vi "Main.vi"() -> ()   [LabVIEW 2018]
uses:
  <vilib>/myRIO/Instrument Drivers/Onboard IO/AI/vis/Read.vi
  <vilib>/myRIO/Common/Instrument Driver Framework/myRIO v1.0/UART/vis/myRIO v1.0 Close UART.vi
  <vilib>/myRIO/Instrument Drivers/Onboard IO/AI/vis/Smart Open.vi
  <vilib>/Utility/error.llb/Error Cluster From Error Code.vi
  <vilib>/myRIO/Common/Instrument Driver Framework/myRIO v1.0/AI/vis/myRIO v1.0 Read AI.vi
  <vilib>/myRIO/Common/Instrument Driver Framework/Utilities/vis/FPGA Ref Manager.vi
  <vilib>/myRIO/Common/Instrument Driver Framework/myRIO v1.0/myRIO v1.0 Reset FPGA.vi
  <vilib>/myRIO/Common/Instrument Driver Framework/myRIO v1.0/IRQ/vis/myRIO v1.0 IRQ Info FGV.vi
  <vilib>/myRIO/Common/Instrument Driver Framework/myRIO v1.0/IRQ/vis/myRIO v1.0 Timer IRQ Info FGV.vi
  <vilib>/myRIO/Common/Instrument Driver Framework/myRIO v1.0/IRQ/vis/myRIO v1.0 ISR Agent.vi
  <vilib>/myRIO/Instrument Drivers/Utilities/Utilities.lvlib
  <vilib>/ptbypt/NI_PtbyPt.lvlib
panel:
  out "웨이브폼 차트":dbl(graph)
  out "범위 밖":bool
  out "numeric":dbl format="%_3g"
  in  "Koffset [cm]":dbl
  in  "Kscale [cm-V]":dbl=27.5
  out "Vo [V]":dbl format="%.2f"
  out "Range [cm]":dbl(knob) scale=0.0..80.0
  in  "[ESC]":bool
  # "IR Range Finder demo"
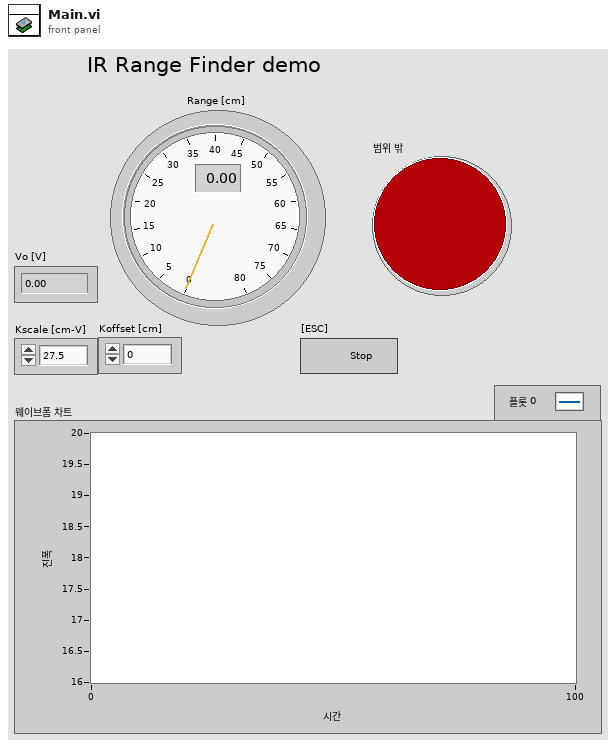
[diagram p1: front panel]
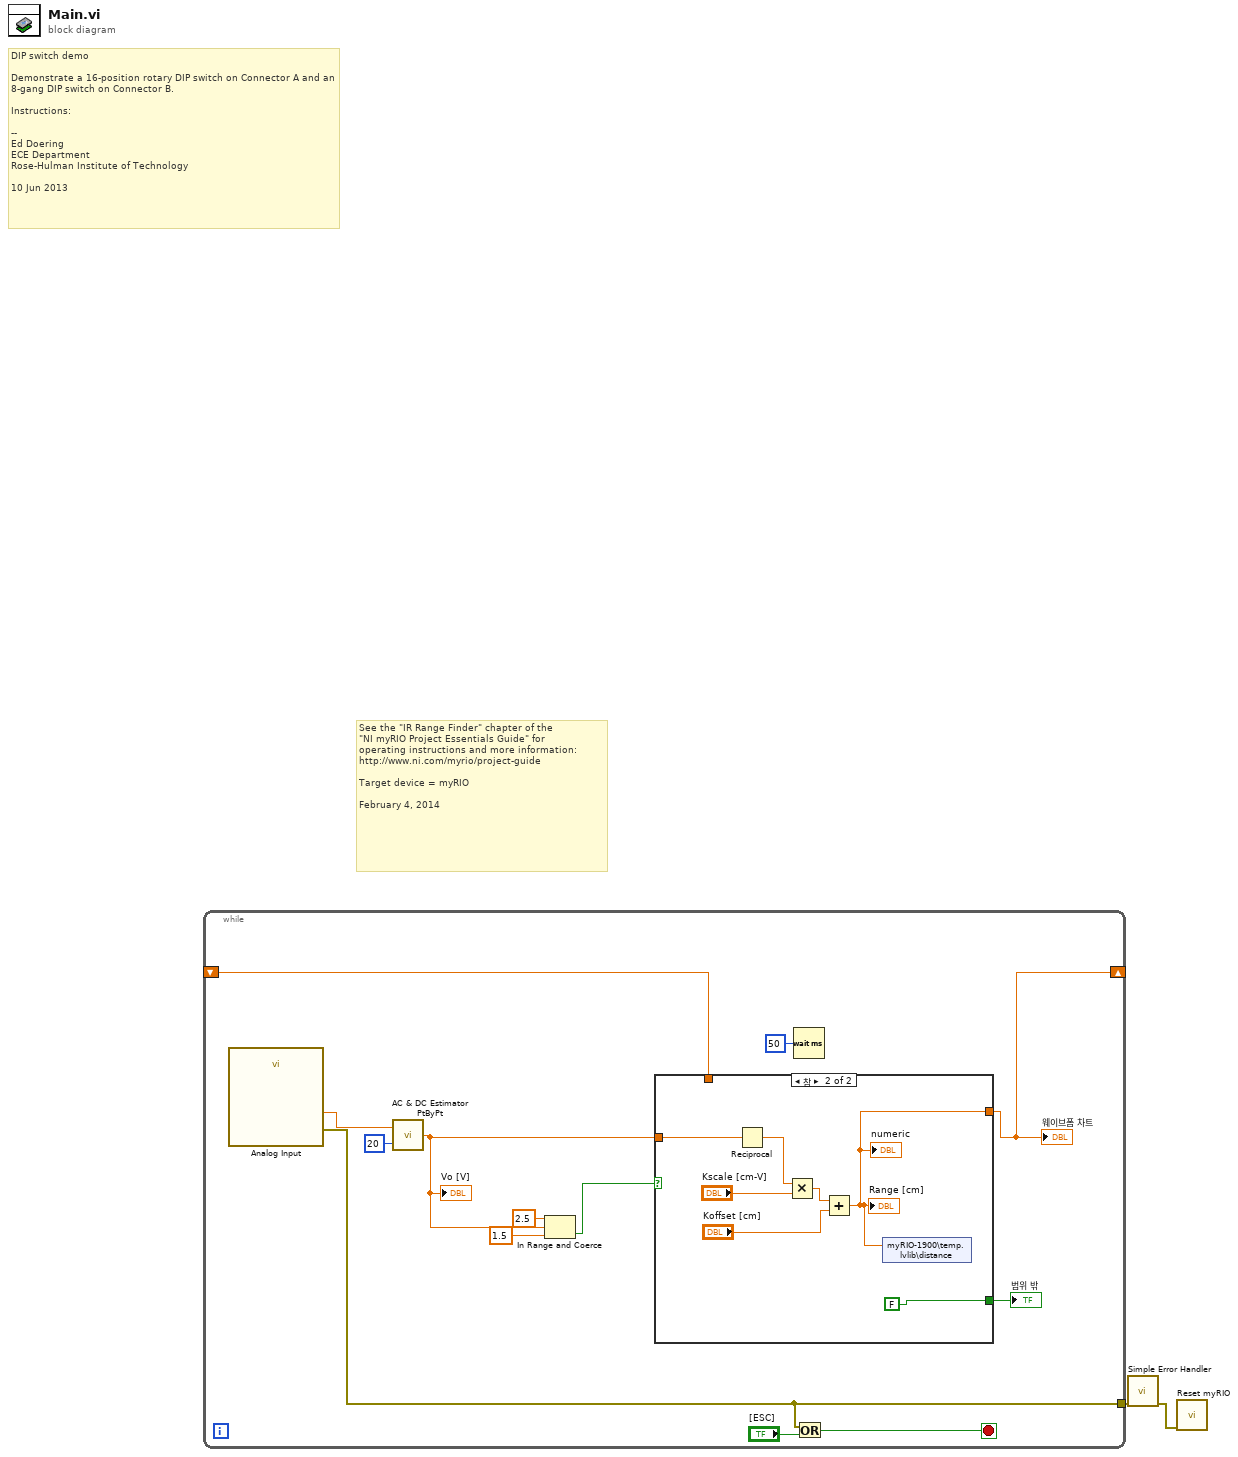
[diagram p0: block diagram]
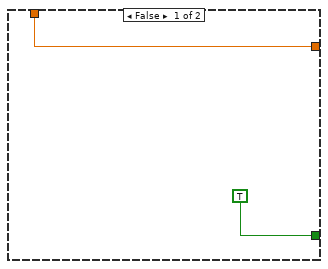
[diagram p2: hidden frame]
diagram:
  # "See the \"IR Range Finder\" chapter of the\n\"NI myRIO Project Essentials Guide\" for\noperating instructions and more information: \nhttp://www.ni.com/myrio/project-guide\n\nTarget device = myRIO\n\nFebruary 4, 2014"
  # "DIP switch demo\n\nDemonstrate a 16-position rotary DIP switch on Connector A and an 8-gang DIP switch on Connector B.\n\nInstructions:\n\n-- \nEd Doering\nECE Department\nRose-Hulman Institute of Technology\n\n10 Jun 2013"
  n1 = while {
    tunnel: [w12] -> w1
    shift-right: [w3] -> _
    shift-left: _ -> [w4]
    stop <- w14 stop-if-true
    n2 = call "Analog Input"() -> ("B/AI0 (Pin 3)"=w11:dbl, "error out"=w12:errorcluster)  [unwired: 26 in]
    n3 = call <vilib>:"AC & DC Estimator PtByPt.vi"("signal"=w11, "sample length"=20) -> ("DC estimate (V)"=w9:dbl)  [unwired: 1 in, 2 out]
    "Vo [V]" <- w9
    n4 = In Range and Coerce(upper limit=2.5 ("상위 리미트"), x=w9, lower limit=1.5 ("하위 리미트")) -> (In Range?=w6:bool)  [unwired: 1 out]
    n5 = case shown="참" w6 {
      tunnel: w9 -> [_ w20]
      tunnel: [TRUE ("범위 밖") FALSE ("범위 밖")] -> w5
      tunnel: w4 -> [w16 _]
      tunnel: [w16 w18] -> w3
      frame False {
      }
      frame True {
        n6 = Reciprocal(x=w20) -> (1/x=w24:dbl)
        n7 = Multiply(x=w24, y="Kscale [cm-V]") -> (x*y=w21:dbl)
        n8 = Add(x=w21, y="Koffset [cm]") -> (x+y=w18:dbl)
        "Range [cm]" <- w18
        "numeric" <- w18
        n9 = shared-variable "myRIO-1900\\temp.lvlib\\distance"(w18) -> ()  [unwired: 1 in, 1 out]
      }
    }
    "범위 밖" <- w5
    "웨이브폼 차트" <- w3
    n10 = Wait (ms)(milliseconds to wait=u32 50) -> ()  [unwired: 1 out]
    n11 = Or(x=w12, y="[ESC]") -> (x .or. y?=w14:bool)
  }
  n12 = call <vilib>:"Simple Error Handler.vi"("error in (no error)"=w1) -> ("error out"=w2:errorcluster)  [unwired: 4 in, 4 out]
  n13 = call <vilib>:"Reset myRIO.vi"("error in (no error)"=w2) -> ()  [unwired: 10 in, 1 out]
